vi "Popout SubPanel.vi"(8 "error in (no error)":errorcluster, 10 "SubPanel":refnum<vi>, 11 "Manager in":refnum<class "Manager.lvclass">) -> (0 "error out":errorcluster, 3 "Manager out":refnum<class "Manager.lvclass">)   [LabVIEW 2020, in "OOPanel.lvlib" / "Manager.lvclass"]
uses:
  Manager.lvclass
  Panel/Panel.lvclass
  Manager.lvclass/Manager.ctl
panel:
  out "Panel":refnum<class "Panel.lvclass">
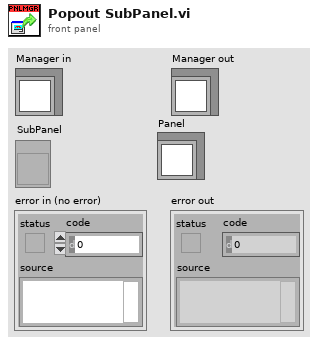
[diagram p1: front panel]
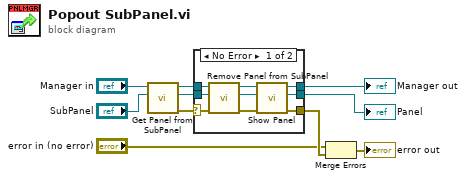
[diagram p0: block diagram]
diagram:
  n1 = call "Get Panel from SubPanel.vi"("SubPanel"="SubPanel", "Manager in"="Manager in") -> ("error out"=w4:errorcluster, "Panel"=w7:refnum<class "Panel.lvclass">, "Manager out"=w8:refnum<class "Manager.lvclass">)  [unwired: 6 in, 1 out]
  n2 = case shown="No Error" w4 {
    selector: w4 -> [w13 w21]
    tunnel: w8 -> [w19 w20]
    tunnel: w7 -> [w18 _]
    tunnel: [w15 w20] -> w6
    tunnel: [w14 _] -> w5
    tunnel: [w11 w21] -> w3
    frame No Error {
      n3 = call "Remove Panel from SubPanel.vi"("error in (no error)"=w13, "Panel In"=w18, "Manager in"=w19) -> ("error out"=w12:errorcluster, "Panel"=w16:refnum<class "Panel.lvclass">, "Manager out"=w17:refnum<class "Manager.lvclass">)  [unwired: 6 in]
      n4 = call "Show Panel.vi"("error in (no error)"=w12, "Panel In"=w16, "Manager in"=w17) -> ("error out"=w11:errorcluster, "Panel"=w14:refnum<class "Panel.lvclass">, "Manager out"=w15:refnum<class "Manager.lvclass">)  [unwired: 6 in]
    }
    frame Error {
    }
  }
  "Manager out" <- w6
  "Panel" <- w5
  n5 = Merge Errors("error in (no error)", w3) -> (→"error out":errorcluster)
